vi "Append text to a file.vi"(8 "Error In":errorcluster, 9 "Overwrite file?":bool, 10 "Text to write to file":string) -> (0 "Error Out":errorcluster, 2 "Contents of Log.txt":string)   [LabVIEW 2013]
doc: "This VI writes the specified string to Log.txt, which is saved in the same folder as this VI.\nIf the user selects the Overwrite boolean control the data in the file is overwritten.\n\nDr. Chris Empson\nSchool of Chemistry\nUniversity of Leeds\nUK\n\nc.j.empson@leeds.ac.uk\nTwitter: @monty_mcmont\nDownloaded from https://github.com/mcmont/LabVIEW_examples"
panel:
  # "Append text to a file.\n\nDr. Chris Empson\nSchool of Chemistry\nUniversity of Leeds\nUK\n\nc.j.empson@leeds.ac.uk\nTwitter: @monty_mcmont\nDownloaded from https://github.com/mcmont/LabVIEW_examples"
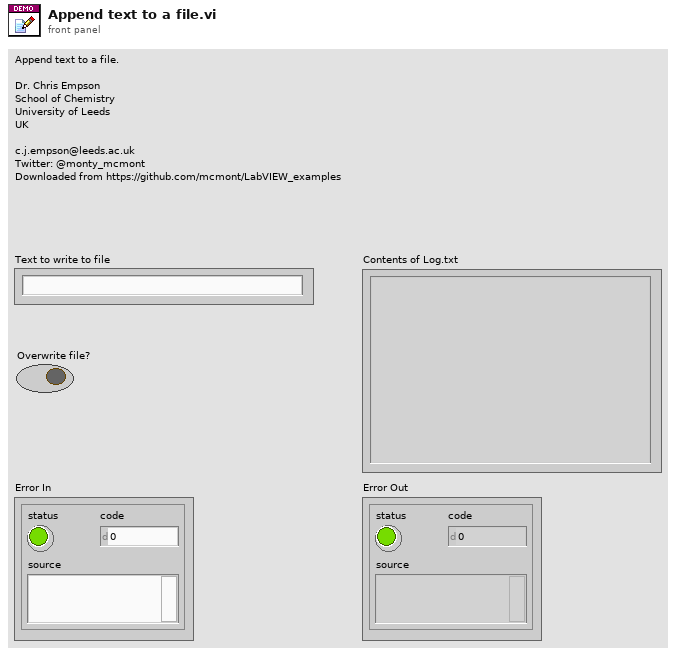
[diagram p1: front panel]
types:
  T1 = enum16{"open", "replace", "create", "open or create", "replace or create", "replace or create with confirmation"}
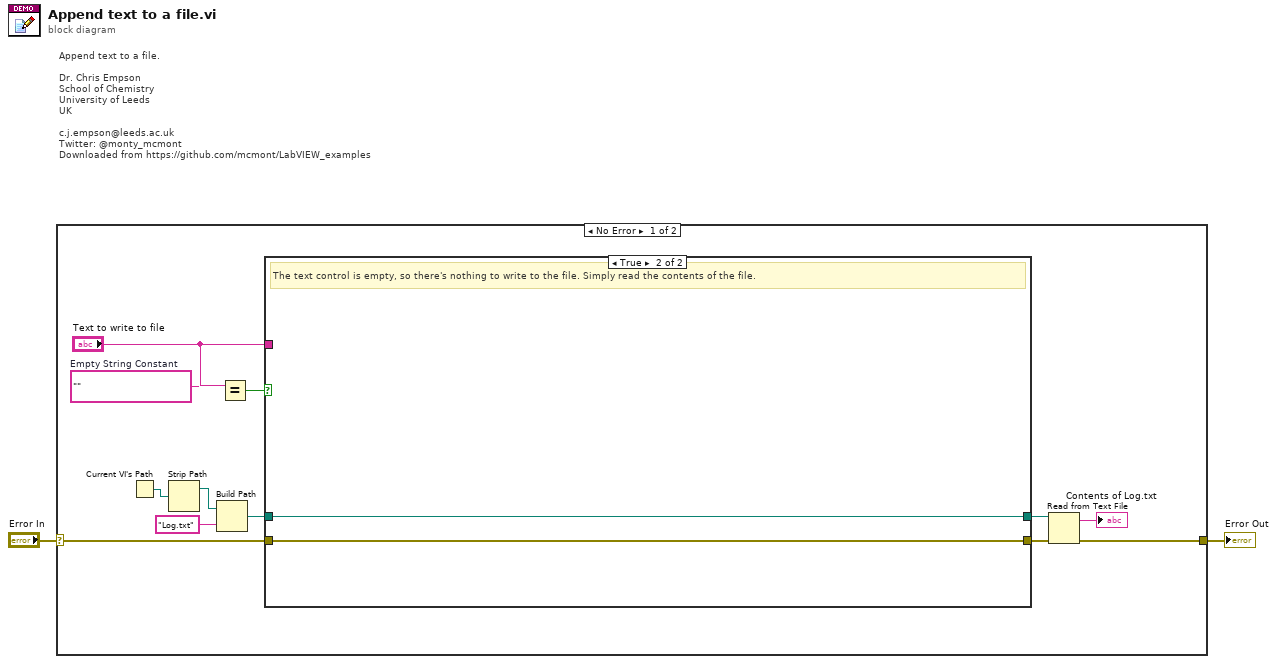
[diagram p0: block diagram]
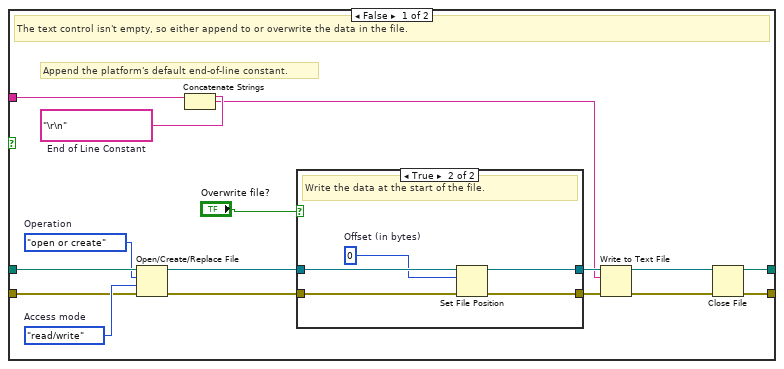
[diagram p2: hidden frame]
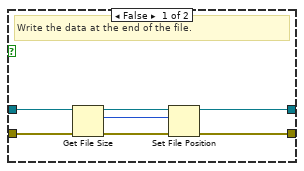
[diagram p3: hidden frame]
diagram:
  # "Append text to a file.\n\nDr. Chris Empson\nSchool of Chemistry\nUniversity of Leeds\nUK\n\nc.j.empson@leeds.ac.uk\nTwitter: @monty_mcmont\nDownloaded from https://github.com/mcmont/LabVIEW_examples"
  n1 = case shown="No Error" "Error In" {
    selector: "Error In" -> [w5 w45]
    tunnel: [w10 w45] -> w1
    frame No Error {
      w3 = ""  # Empty String Constant
      n2 = Current VI's Path() -> (path=w14:path)
      n3 = Strip Path(path=w14) -> (stripped path=w6:path)  [unwired: 1 out]
      n4 = Build Path(base path=w6, name or relative path="Log.txt") -> (appended path=w12:path)
      n5 = Equal?(x="Text to write to file", y=w3) -> (x = y?=w7:bool)
      n6 = case shown="True" w7 {
        tunnel: w12 -> [w30 w44]
        tunnel: [w20 w44] -> w11
        tunnel: [w19 w43] -> w9
        tunnel: w5 -> [w18 w43]
        tunnel: "Text to write to file" -> [w16 _]
        frame False {
          w17 = "\r\n"  # End of Line Constant
          w26 = enum16{"read/write", "read-only", "write-only"}."read/write"  # Access mode
          w29 = T1."open or create"  # Operation
          # "Append the platform's default end-of-line constant."
          # "The text control isn't empty, so either append to or overwrite the data in the file."
          n7 = Open/Create/Replace File(file path (use dialog)=w30, error in=w18, operation (0:open)=w29, access (0:read/write)=w26) -> (refnum out=w24:refnum<file>, error out=w25:errorcluster)  [unwired: 2 in, 1 out]
          n8 = Concatenate Strings(w16, w17) -> (w15:string)
          n9 = case shown="True" "Overwrite file?" {
            tunnel: w25 -> [w31 w41]
            tunnel: w24 -> [w37 w42]
            tunnel: [w35 w39] -> w23
            tunnel: [w34 w40] -> w22
            frame False {
              # "Write the data at the end of the file."
              n10 = Get File Size(file=w37, error in=w31) -> (refnum out=w36:refnum<file>, size (in bytes)=w32:i64, 0:w33:errorcluster)
              n11 = Set File Position(offset (in bytes) (0)=w32, refnum=w36, error in=w33) -> (refnum out=w35:refnum<file>, error out=w34:errorcluster)  [unwired: 1 in]
            }
            frame True {
              w38 = i64 0  # Offset (in bytes)
              # "Write the data at the start of the file."
              n12 = Set File Position(offset (in bytes) (0)=w38, refnum=w42, error in=w41) -> (refnum out=w39:refnum<file>, error out=w40:errorcluster)  [unwired: 1 in]
            }
          }
          n13 = Write to Text File(file (use dialog)=w23, text=w15, error in=w22) -> (refnum out=w28:refnum<file>, error out=w27:errorcluster)  [unwired: 1 in, 1 out]
          n14 = Close File(refnum=w28, error in=w27) -> (path=w20:path, error out=w19:errorcluster)
        }
        frame True {
          # "The text control is empty, so there's nothing to write to the file. Simply read the contents of the file."
        }
      }
      n15 = Read from Text File(file (use dialog)=w11, error in=w9) -> (text=→"Contents of Log.txt":string, error out=w10:errorcluster)  [unwired: 2 in, 2 out]
    }
    frame Error {
    }
  }
  "Error Out" <- w1
